vi "Vibration.vi"() -> ()   [LabVIEW 2012]
panel:
  out "?":enum32{"选项卡 1", "选项卡 2"}(tab)
  in  "配置":bool
  in  "AC/DC":bool
  in  "开始":bool
  in  "采样率(ksps)":T1(ring)=enum."105.468"
  in  "装置IP":string="192.168.1.16"
  in  "灵敏度4(mv/g)":i32=1 min=1
  in  "灵敏度3(mv/g)":i32=1 min=1
  in  "灵敏度2(mv/g)":i32=1 min=1
  in  "灵敏度1(mv/g)":i32=1 min=1
  in  "通道4":bool=TRUE
  in  "通道3":bool=TRUE
  in  "通道2":bool=TRUE
  in  "通道1":bool=TRUE
  out "?":dbl[][](graph)
  out "?":u16[](graph)
  in  "是否开启电流源":bool=TRUE
  in  "是否进行自校准":bool
  in  "是否保存数据":bool
  in  "保存路径":path
  in  "设置装置IP":string="192.168.1.16"
  in  "设置装置子网掩码":string="255.255.255.0"
  in  "设置装置网关":string="192.168.1.1"
  in  "?":bool
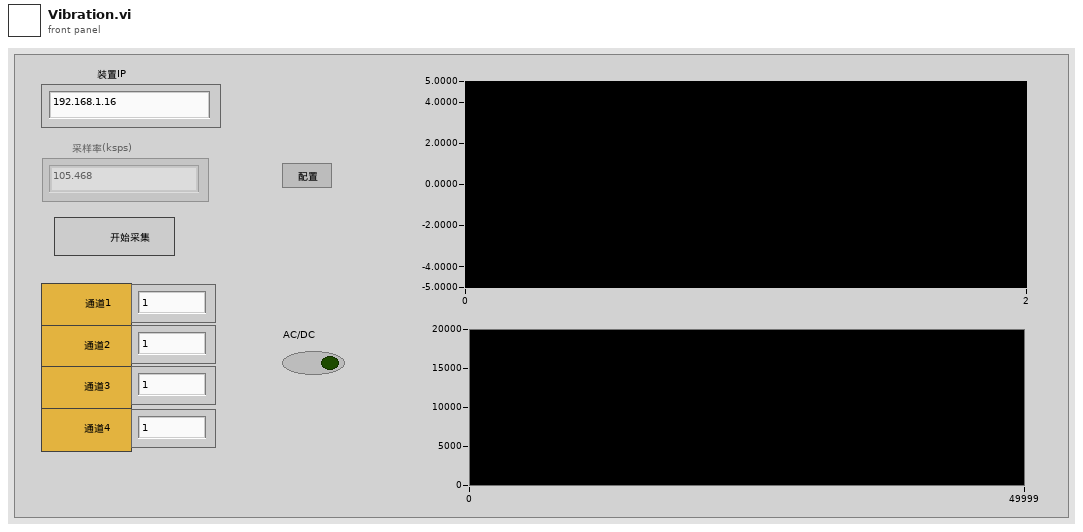
[diagram p1: front panel]
types:
  T1 = enum16{"", "105.468", "52.734", "35.156", "26.367", "21.094", "17.578", "15.067", "13.184", "11.719", "10.545"}
  T2 = enum8{"Enabled", "Disabled", "Disabled and Grayed Out"}
  T3 = cluster{"refnum":refnum<file>, "refnum":refnum<file>, "refnum":refnum<file>, "refnum":refnum<file>, "refnum":refnum<file>, "SavePath":path, "SAVE?":bool, "connection ID":refnum<k5>}
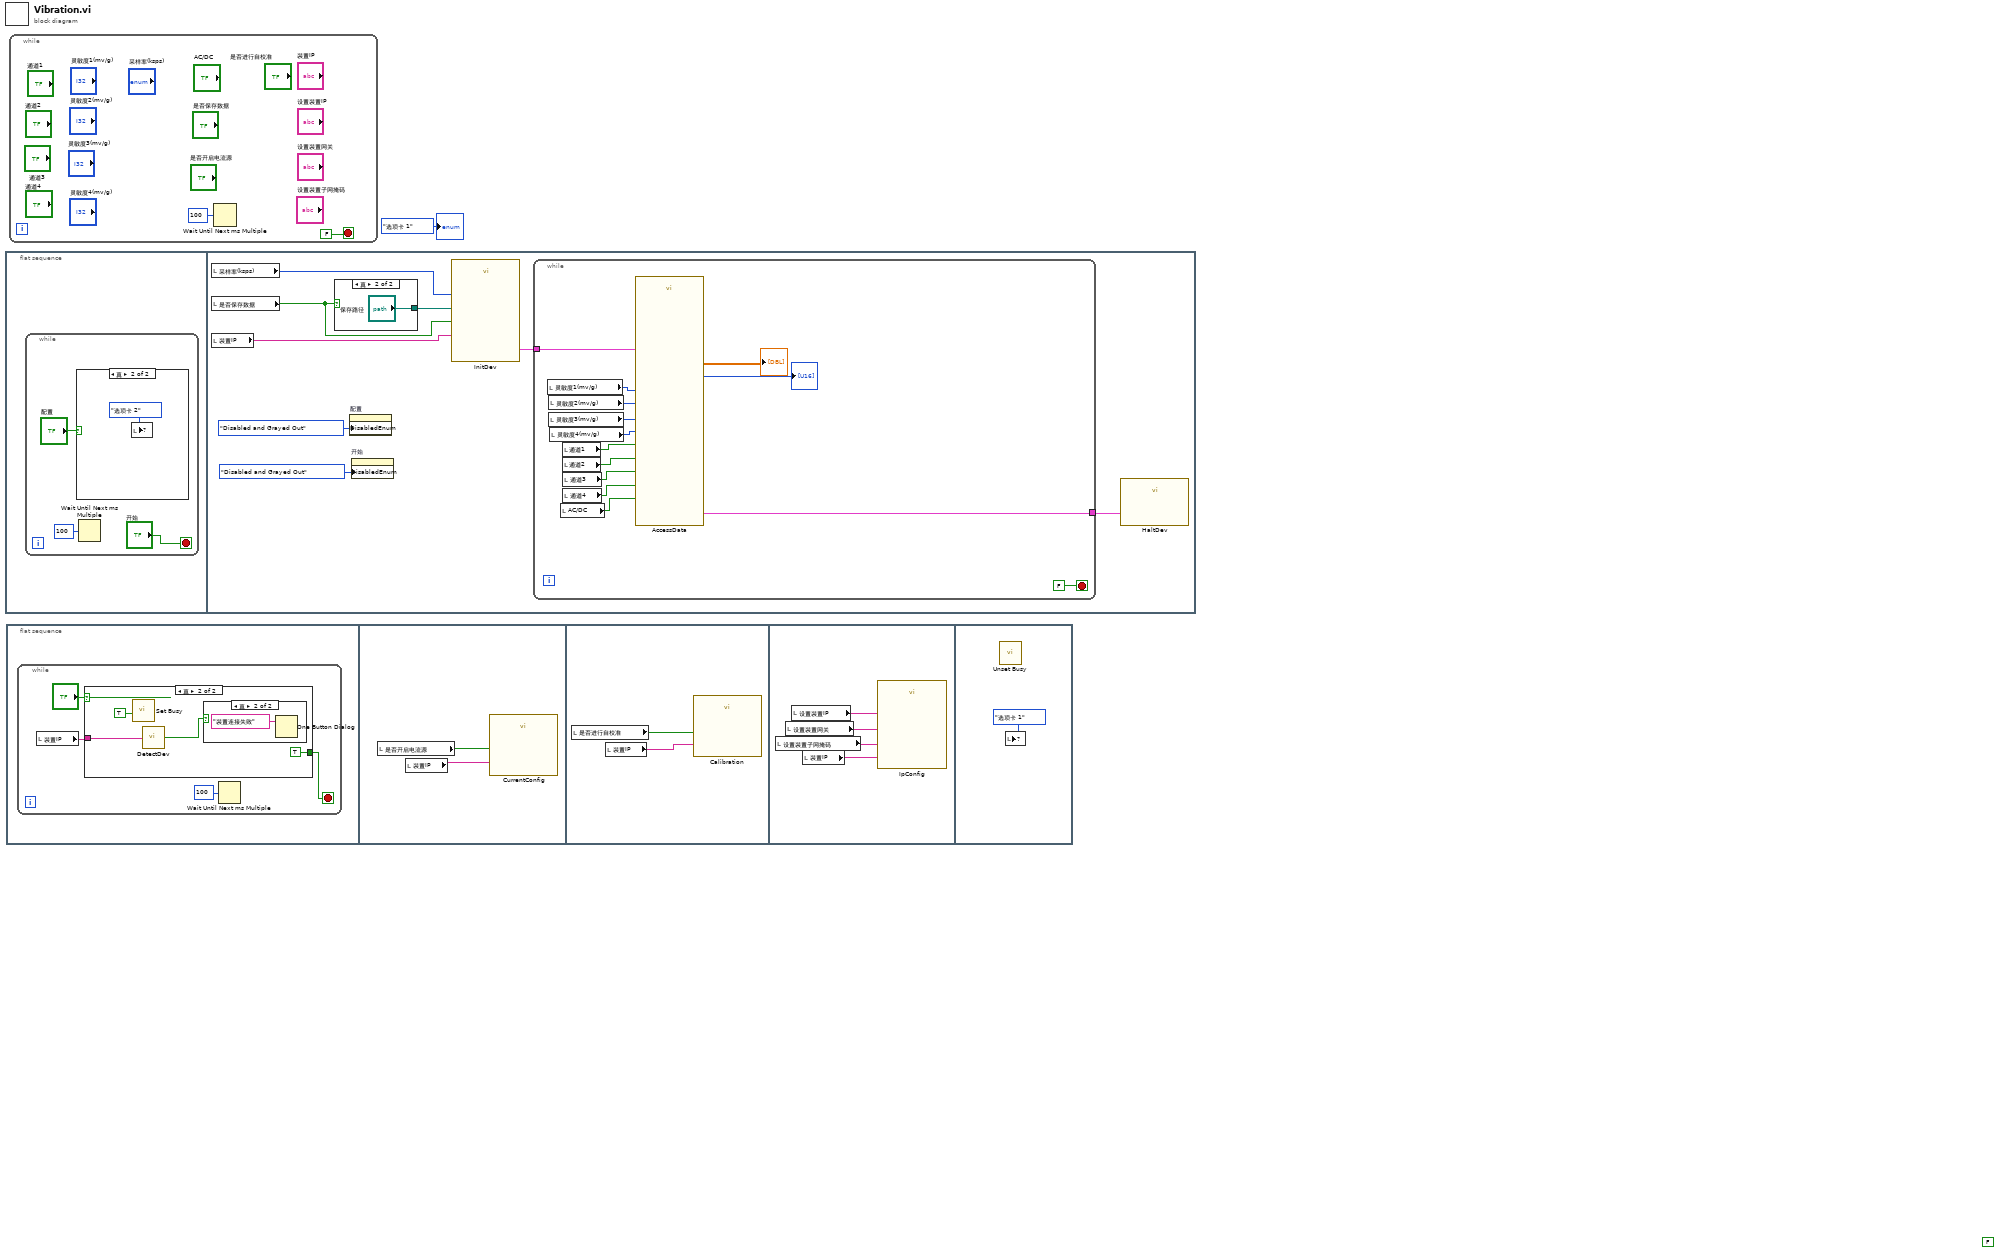
[diagram p0: block diagram]
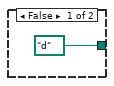
[diagram p3: hidden frame]
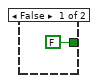
[diagram p4: hidden frame]
diagram:
  (unwired) FALSE
  n1 = flat-sequence {
    frame #0 {
      n2 = while {
        stop <- "开始" stop-if-true
        n3 = case shown="真" "配置" {
          frame False {
          }
          frame True {
            n4 = local write item#21(enum32{"选项卡 1", "选项卡 2"}."选项卡 2" ("选项卡控件")) -> ()
          }
        }
        n5 = Wait Until Next ms Multiple(millisecond multiple=u32 100 ("毫秒倍数")) -> ()  [unwired: 1 out]
      }
    }
    frame #1 {
      n6 = local read "采样率(ksps)"() -> (w12:T1)
      n7 = local read "是否保存数据"() -> (w13:bool)
      n8 = local read "装置IP"() -> (w9:string)
      n9 = case shown="真" w13 {
        tunnel: [path "d:/" ("路径（使用对话框）") "保存路径"] -> w8
        frame False {
        }
        frame True {
        }
      }
      n10 = property on="配置" class="Bool"("DisabledEnum"=T2."Disabled and Grayed Out" ("禁用")) -> ()  [unwired: 2 in, 2 out]
      n11 = property on="开始" class="Bool"("DisabledEnum"=T2."Disabled and Grayed Out" ("禁用")) -> ()  [unwired: 2 in, 2 out]
      n12 = call "InitDev.vi"("SAVE?"=w13, "IP地址"=w9, "SampleRate"=w12, "SavePath"=w8) -> ("输出簇"=w10:T3)
      n13 = while {
        tunnel: w10 -> [w27]
        tunnel: [w26] -> w11
        stop <- FALSE stop-if-true
        n14 = local read "灵敏度1(mv/g)"() -> (w23:i32)
        n15 = local read "灵敏度2(mv/g)"() -> (w22:i32)
        n16 = local read "灵敏度3(mv/g)"() -> (w21:i32)
        n17 = local read "灵敏度4(mv/g)"() -> (w20:i32)
        n18 = local read "AC/DC"() -> (w15:bool)
        n19 = local read "通道1"() -> (w19:bool)
        n20 = local read "通道2"() -> (w18:bool)
        n21 = local read "通道3"() -> (w17:bool)
        n22 = local read "通道4"() -> (w16:bool)
        n23 = call "AccessData.vi"("Sensitivity1"=w23, "CH1Enable"=w19, "Sensitivity2"=w22, "CH2Enable"=w18, "Sensitivity3"=w21, "CH3Enable"=w17, "Sensitivity4"=w20, "CH4Enable"=w16, "输入簇"=w27, "RmOffset"=w15) -> ("VibrationWave"=→"?":dbl[][], "Speed"=→"?":u16[], "输出簇"=w26:T3)  [unwired: 2 in, 1 out]
      }
      n24 = call "HaltDev.vi"("输入簇"=w11) -> ()
    }
  }
  n25 = flat-sequence {
    frame #0 {
      n26 = while {
        stop <- w32 stop-if-true
        n27 = local read "装置IP"() -> (w30:string)
        n28 = case shown="真" "?" {
          tunnel: [FALSE TRUE] -> w32
          tunnel: w30 -> [_ w37]
          frame False {
          }
          frame True {
            n29 = call <vilib>:"Set Busy.vi"("disable click? (T)"=TRUE) -> ()  [unwired: 9 in, 2 out]
            n30 = call "DetectDev.vi"("IP."=w37) -> ("Fail"=w38:bool)
            n31 = case shown="真" w38 {
              frame False {
              }
              frame True {
                n32 = One Button Dialog(message="装置连接失败" ("消息")) -> ()  [unwired: 1 in, 1 out]
              }
            }
          }
        }
        n33 = Wait Until Next ms Multiple(millisecond multiple=u32 100 ("毫秒倍数")) -> ()  [unwired: 1 out]
      }
    }
    frame #1 {
      n34 = local read "是否开启电流源"() -> (w40:bool)
      n35 = local read "装置IP"() -> (w41:string)
      n36 = call "CurrentConfig.vi"("Current"=w40, "IP"=w41) -> ()
    }
    frame #2 {
      n37 = local read "是否进行自校准"() -> (w43:bool)
      n38 = local read "装置IP"() -> (w42:string)
      n39 = call "Calibration.vi"("Enable"=w43, "IP."=w42) -> ()
    }
    frame #3 {
      n40 = local read "设置装置子网掩码"() -> (w45:string)
      n41 = local read "设置装置网关"() -> (w46:string)
      n42 = local read "设置装置IP"() -> (w47:string)
      n43 = local read "装置IP"() -> (w44:string)
      n44 = call "IpConfig.vi"("Gateway"=w46, "SubnetMask"=w45, "IP"=w47, "CurrentIP"=w44) -> ()
    }
    frame #4 {
      n45 = call <vilib>:"Unset Busy.vi"() -> ()  [unwired: 11 in, 1 out]
      n46 = local write item#21(enum32{"选项卡 1", "选项卡 2"}."选项卡 1" ("选项卡控件")) -> ()
    }
  }
  n47 = while {
    stop <- FALSE stop-if-true
    n48 = Wait Until Next ms Multiple(millisecond multiple=u32 100 ("毫秒倍数")) -> ()  [unwired: 1 out]
  }
  "?" <- enum32{"选项卡 1", "选项卡 2"}."选项卡 1" ("选项卡控件")
